vi "Get Digital Configuration.vi"(8 "error in (no error)":errorcluster, 9 "Digital Index":i32, 10 "PMU Index":i32, 11 "Pseudo PDC ID":i32) -> (0 "error out":errorcluster, 2 "Digital Name":string, 3 "Digital Configuration":cluster{"normalBit":u8, "isValidBit":u8})   [LabVIEW 2013, in "PMU Recorder Light.lvlib" / "Statnett C37.118 DLL.lvclass"]
uses:
  Statnett C37.118 DLL.lvclass
  c37118-dll/C37118-DLL.lvlib
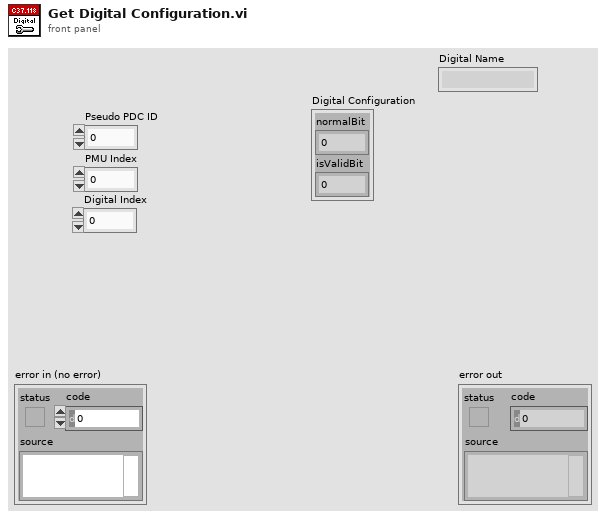
[diagram p1: front panel]
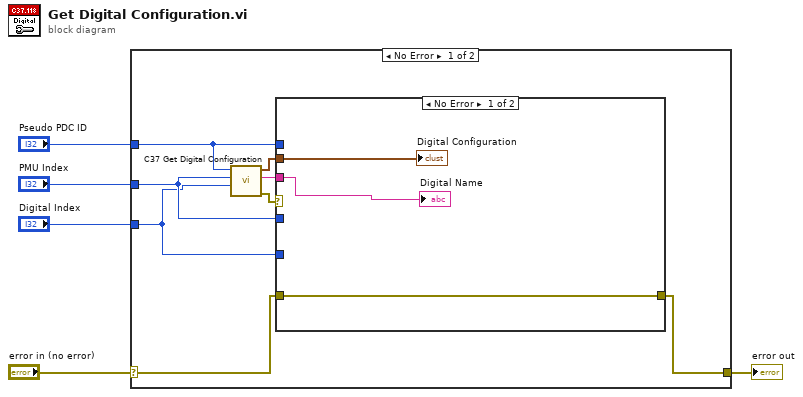
[diagram p0: block diagram]
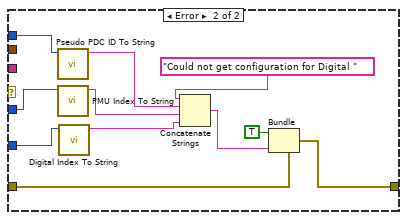
[diagram p2: hidden frame]
diagram:
  n1 = case shown="No Error" "error in (no error)" {
    selector: "error in (no error)" -> [w13 w28]
    tunnel: [w12 w28] -> w4
    tunnel: "Pseudo PDC ID" -> [w8 _]
    tunnel: "PMU Index" -> [w7 _]
    tunnel: "Digital Index" -> [w6 _]
    frame No Error {
      n2 = call "C37 Get Digital Configuration.vi"("Digital Index"=w6, "PMU Index"=w7, "Pseudo PDC ID"=w8) -> ("error out"=w11:errorcluster, "Channel Name"=w9:string, "Digital Configuration"=w10:cluster{"normalBit":u8, "isValidBit":u8})  [unwired: 6 in]
      n3 = case shown="No Error" w11 {
        tunnel: w13 -> [w16 w27]
        tunnel: w7 -> [_ w21]
        tunnel: [w16 w23] -> w12
        tunnel: w10 -> [w15 _]
        tunnel: w9 -> [w14 _]
        tunnel: w8 -> [_ w22]
        tunnel: w6 -> [_ w18]
        frame No Error {
          "Digital Name" <- w14
          "Digital Configuration" <- w15
        }
        frame Error {
          n4 = call "Pseudo PDC ID To String.vi"("Pseudo PDC ID"=w22) -> ("String"=w20:string)  [unwired: 10 in]
          n5 = call "PMU Index To String.vi"("PMU Index"=w21) -> ("String"=w19:string)  [unwired: 10 in]
          n6 = call "Digital Index To String.vi"("Digital Index"=w18) -> ("String"=w17:string)  [unwired: 10 in]
          n7 = Concatenate Strings("Could not get configuration for Digital " ("source"), w20, w19, w17) -> (w24:string)
          n8 = Bundle(cluster=w27, "status"=TRUE, "source"=w24) -> (w23:errorcluster)  [unwired: 1 in]
        }
      }
    }
    frame Error {
    }
  }
  "error out" <- w4
